vi "CreateGradTable.vi"(10 "Count by Class":i32[](array[numeric])=[0, 0, 0, 0], 11 "Freshmen Graduation Year":i8) -> (3 "Combined Grad Table":string)   [LabVIEW 2015]
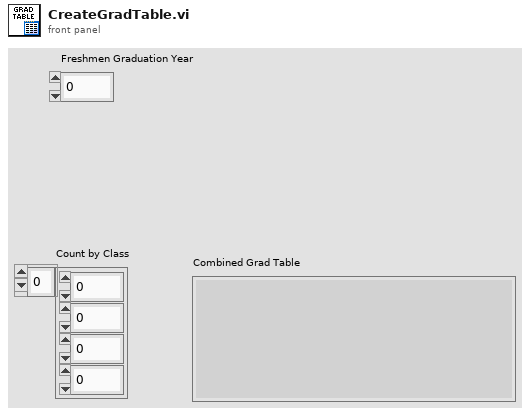
[diagram p1: front panel]
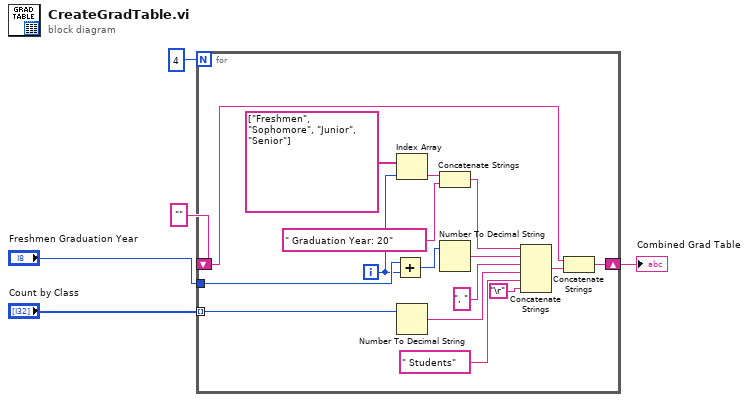
[diagram p0: block diagram]
diagram:
  n1 = for {
    N: 4 -> [_]
    tunnel: "Freshmen Graduation Year" -> [w16]
    tunnel: "Count by Class" -> [w12] mode=indexing
    shift-right: [w6] -> w2
    shift-left: "" -> [w8]
    i -> [w15]
    n2 = Add(x=w16, y=w15) -> (x+y=w14:i32)
    n3 = Index Array(array=string[] ["Freshmen", "Sophomore", "Junior", "Senior"], index=w15) -> (element=w20:string)
    n4 = Number To Decimal String(number=w12) -> (decimal integer string=w11:string)  [unwired: 1 in]
    n5 = Concatenate Strings(w20, " Graduation Year: 20" ("string")) -> (w17:string)
    n6 = Number To Decimal String(number=w14) -> (decimal integer string=w18:string)  [unwired: 1 in]
    n7 = Concatenate Strings(w17, w18, ", " ("string"), w11, " Students" ("string"), "\r") -> (w7:string)
    n8 = Concatenate Strings(w8, w7) -> (w6:string)
  }
  "Combined Grad Table" <- w2
